vi "Exchange Param.vi"(4 "PAR index":u16[](array[numeric]), 6 "PAR":dbl[](array[numeric]), 8 "error in (no error)":errorcluster, 9 "AOP index":u16[](array[numeric]), 10 "AOP":dbl[][](array[numeric]), 11 "Regs":refnum<class "bronkhorst_reg.lvclass">[](array[class])) -> (0 "error out":errorcluster, 3 "Regs out":refnum<class "bronkhorst_reg.lvclass">[](array[class]))   [LabVIEW 2019, in "bronkhorst_reg.lvclass"]
uses:
  bronkhorst_reg.lvclass
  ctl/control param.ctl
  bronkhorst_reg.lvclass/bronkhorst_reg.ctl
  control.lvlib
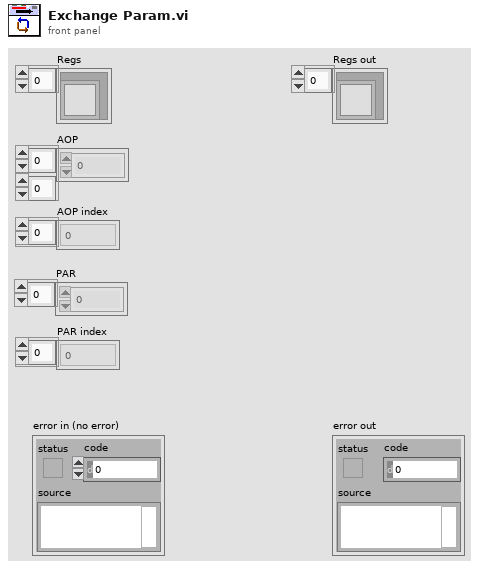
[diagram p1: front panel]
types:
  T1 = typedef "control.lvlib/control param.ctl" = cluster{"proportional gain (Kc)":dbl, "integral time (Ti, s)":dbl, "derivative time (Td, s)":dbl, "output high":dbl, "output high start":dbl, "output high stop":dbl, "alr value":dbl, "output low":dbl, "output rate (EGU/s)":dbl, "setpoint max":dbl, "setpoint rate (EGU/min)":dbl, "stop rate (EGU/min)":dbl}
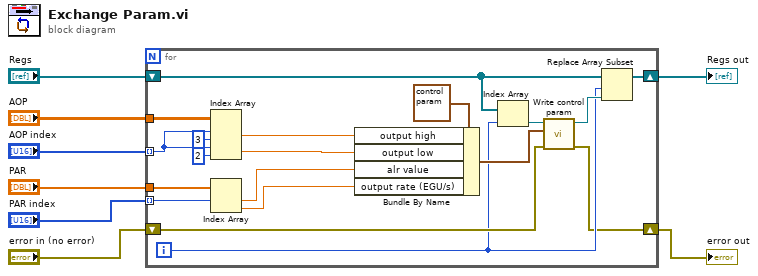
[diagram p0: block diagram]
diagram:
  n1 = for {
    tunnel: "AOP" -> [w27]
    tunnel: "PAR" -> [w26]
    tunnel: "PAR index" -> [w25] mode=indexing
    shift-right: [w17] -> w7
    shift-left: "Regs" -> [w16]
    shift-right: [w12] -> w2
    shift-left: "error in (no error)" -> [w14]
    tunnel: "AOP index" -> [w9] mode=indexing
    i -> [w13]
    n2 = Index Array(array=w27, index (row) #1=w9, index (col) #1=3 ("index"), index (row) #2=w9, index (col) #2=2 ("index")) -> (element #1=w23:dbl, element #2=w22:dbl)
    n3 = Index Array(array=w26, index #1=w25) -> (element #1=w21:dbl, element #2=w20:dbl)  [unwired: 1 in]
    n4 = Bundle By Name(cluster=T1 {"proportional gain (Kc)"=1.0, "integral time (Ti, s)"=10.0, "derivative time (Td, s)"=1.0, "output high"=100.0, "output high start"=40.0, "output high stop"=40.0, "alr value"=0.0, "output low"=0.0, "output rate (EGU/s)"=5.0, "setpoint max"=100.0, "setpoint rate (EGU/min)"=10.0, "stop rate (EGU/min)"=5.0} ("control param"), "output high"=w23, "output low"=w22, "alr value"=w21, "output rate (EGU/s)"=w20) -> (w18:T1)
    n5 = Index Array(array=w16, index=w13) -> (element=w19:refnum<class "bronkhorst_reg.lvclass">)
    n6 = call "Write control param.vi"("error in (no error)"=w14, "control param"=w18, "reg in"=w19) -> ("error out"=w12:errorcluster, "reg out"=w15:refnum<class "bronkhorst_reg.lvclass">)  [unwired: 7 in]
    n7 = Replace Array Subset(array=w16, new element=w15, index=w13) -> (w17:refnum<class "bronkhorst_reg.lvclass">[])
  }
  "error out" <- w2
  "Regs out" <- w7
